vi "Render.vi"(8 "error in (no error)":errorcluster, 10 "String in":string, 11 "OrderedList in":refnum<class "TaskList.lvclass">) -> (0 "error out":errorcluster, 2 "String out":string, 3 "OrderedList out":refnum<class "TaskList.lvclass">)   [LabVIEW 2021, in "LvMarkdown.lvlib" / "TaskList.lvclass"]
uses:
  TaskList.lvclass
  TaskList.lvclass/TaskList.ctl
  Collection/GetElements.vi
  IRenderable/IRenderable.lvclass
  Collection/Collection.lvclass
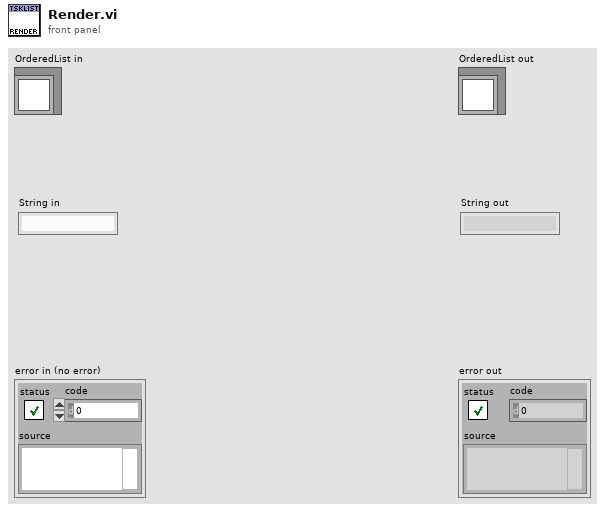
[diagram p1: front panel]
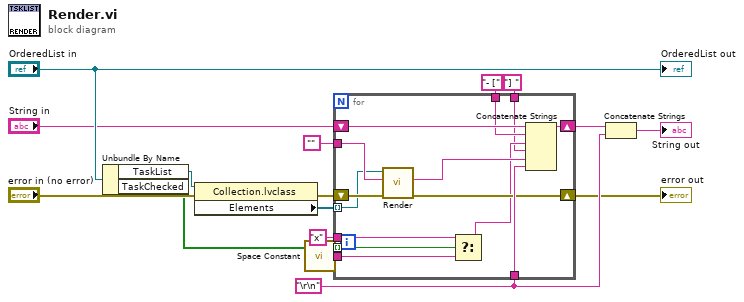
[diagram p0: block diagram]
diagram:
  w12 = "\r\n"
  n1 = Unbundle By Name("OrderedList in") -> ("TaskList"=w15:refnum<class "Collection.lvclass">, "TaskChecked"=w4:bool[])
  n2 = property class="Collection.lvclass"(reference=w15, error in="error in (no error)") -> (error out=w6:errorcluster, "Elements"=w5:refnum<class "IRenderable.lvclass">[])  [unwired: 1 out]
  n3 = call <vilib>:"Space Constant.vi"() -> ("String"=w2:string)
  n4 = for {
    shift-right: [w29] -> w13
    shift-left: "String in" -> [w30]
    tunnel: w12 -> [w28]
    tunnel: "" -> [w26]
    shift-right: [w25] -> w9
    shift-left: w6 -> [w27]
    tunnel: "- [" ("format string") -> [w23]
    tunnel: w5 -> [w24] mode=indexing
    tunnel: w4 -> [w21] mode=indexing
    tunnel: "] " ("string") -> [w19]
    tunnel: w2 -> [w18]
    tunnel: "x" -> [w17]
    n5 = call-dynamic "Render.vi"("error in (no error)"=w27, "String in"=w26, "IRenderable in"=w24) -> ("error out"=w25:errorcluster, "String out"=w22:string)  [unwired: 6 in, 1 out]
    n6 = Select(t=w17, s=w21, f=w18) -> (s? t:f=w20:string)
    n7 = Concatenate Strings(w30, w23, w20, w19, w22, w28) -> (w29:string)
  }
  "error out" <- w9
  n8 = Concatenate Strings(w13, w12) -> (→"String out":string)
  "OrderedList out" <- "OrderedList in"
